vi "PH_BlackBox.constructor.vi"(0 "name":string, 2 "data in":string, 5 "error in(no error)":errorcluster) -> (14 "i ref out":refnum<vi>, 16 "data out":string, 19 "error out":errorcluster)   [LabVIEW 2014, in "PH_BlackBox.lvlib"]
doc: "This class is forseen to control black boxes (motion).\n\nThis class is part of the PHELIX device layer.\n\nauthor: Stefan Götte, GSI\n\nLicense Agreement for this software:\n\nCopyright (C)\nGesellschaft für Schwerionenforschung, GSI\nPlanckstr. 1\n64291 Darmstadt\nGermany\n\nContact: D.Beck@gsi.de \n\nThis program is free software; you can redistribute it and/or modify it under the terms of the \nGNU General Public License as published by the Free Software Foundation; either version 2 of \nthe license, or (at your option) any later version.\n\nThis program is distributed in the hope that it will be useful, but WITHOUT ANY WARRANTY; \nwithout even the implied warranty of MERCHANTABILITY or FITNESS FOR A PARTICULAR PURPOSE. See the GNU General License for more details (http://www.gnu.org).\n\nGesellschaft für Schwerionenforschung, GSI\nPlanckstr. 1, 64291 Darmstadt, Germany\nFor all questions and ideas contact: M.Richter@gsi.de, H.Brand@gsi.de or D.Beck@gsi.de.\nLast update: 16-JUN-2004"
uses:
  PH_BlackBox.lvlib
  PH_Basics/PH_Class/PH_Class.lvlib
  CS_Core/CSSystem/CSSystemLib/CSSystemLib.lvlib
  PH_Basics/PH_PSDBWriter/PH_PSDBWriter.lvlib
  PH_Basics/PH_StatusHandler/PH_StatusHandler.lvlib
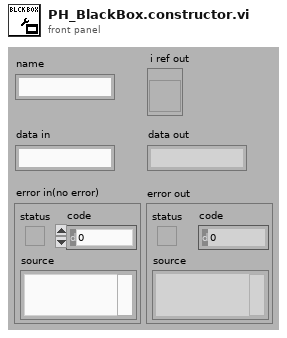
[diagram p1: front panel]
types:
  T1 = enum16{"SetAttribute", "GetAttribute", "CreateAttribute", "DestroyAttribute", "DestroyAllAtributes"}
  T2 = typedef "PH_BlackBox.lvlib/PH_BlackBox.i attribute.ctl" = cluster{"BB Remote Controlled?":bool, "GUI Refs":T3, "Position IN":T4, "Position OUT":T4, "BB Remote Controlled by other Instance?":bool, "Recipient":string, "Number":i32, "Caption Move":string, "Caption Out":string, "Caption In":string}
  T3 = typedef "PH_BlackBox.lvlib/PH_BlackBox.GUI Refs.ctl" = cluster{"MOVE IN":refnum<vi>, "MOVE":refnum<vi>, "IN":refnum<vi>, "OUT":refnum<vi>, "REMOTE":refnum<vi>, "GUI-Knob Move":refnum<vi>, "GUI-Knob Move in":refnum<vi>, "POWER ON":refnum<vi>, "Delete":refnum<vi>, "Function Textfield":refnum<vi>}
  T4 = typedef "PH_StatusHandler.lvlib/PH_StatusHandler.Status.ctl" = i16
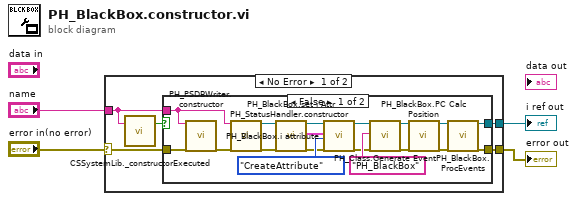
[diagram p0: block diagram]
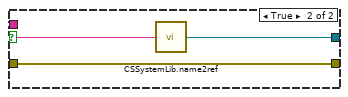
[diagram p2: hidden frame]
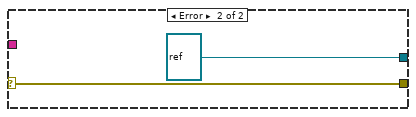
[diagram p3: hidden frame]
diagram:
  n1 = case shown="No Error" "error in(no error)" {
    selector: "error in(no error)" -> [w9 w32]
    tunnel: [w8 refnum<vi> refnum ("i ref out")] -> w4
    tunnel: [w7 w32] -> w3
    tunnel: "name" -> [w6 _]
    frame No Error {
      n2 = call "CSSystemLib._constructorExecuted.vi"("name"=w6) -> ("constructor executed?"=w5:bool)  [unwired: 18 in]
      n3 = case shown="False" w5 {
        tunnel: w9 -> [w13 w30]
        tunnel: [w23 w28] -> w8
        tunnel: [w22 w30] -> w7
        tunnel: w6 -> [w10 w29]
        frame False {
          n4 = call "PH_PSDBWriter.constructor.vi"("name"=w10, "error in"=w13) -> ("error out"=w20:errorcluster)  [unwired: 15 in, 2 out]
          n5 = call "PH_StatusHandler.constructor.vi"("name"=w10, "error in(no error)"=w20) -> ("i ref out"=w11:refnum<vi>, "error out"=w12:errorcluster)  [unwired: 15 in, 1 out]
          n6 = call "PH_BlackBox.set i Attr.vi"("VI in"=w11, "error in (no error)"=w12) -> ("VI out"=w25:refnum<vi>, "i Attribute"=w26:T2, "error out"=w24:errorcluster)  [unwired: 15 in]
          n7 = call "PH_BlackBox.i attribute.vi"("VI Refnum"=w25, "CLASS.i attribute"=w26, "Action"=T1."CreateAttribute", "error in (no error)"=w24) -> ("VI Refnum out"=w17:refnum<vi>, "error out"=w15:errorcluster)  [unwired: 13 in, 1 out]
          n8 = call "PH_Class.Generate Event.vi"("i ref in"=w17, "Class"="PH_BlackBox", "error in (no error)"=w15) -> ("i ref out"=w16:refnum<vi>, "error out"=w14:errorcluster)  [unwired: 15 in]
          n9 = call "PH_BlackBox.PC Calc Position.vi"("i ref in"=w16, "error in (no error)"=w14) -> ("i ref out"=w18:refnum<vi>, "error out"=w19:errorcluster)  [unwired: 16 in]
          n10 = call "PH_BlackBox.ProcEvents.vi"("i ref in"=w18, "error in (no error)"=w19) -> ("i ref out"=w23:refnum<vi>, "error out"=w22:errorcluster)  [unwired: 16 in]
        }
        frame True {
          n11 = call "CSSystemLib.name2ref.vi"("name"=w29) -> ("obj refnum"=w28:refnum<vi>)
        }
      }
    }
    frame Error {
    }
  }
  "i ref out" <- w4
  "error out" <- w3
